vi "Run Program.vi"(0 "Program Path":path=path "%SystemRoot%/System32/calc.exe") -> ()   [LabVIEW 2020]
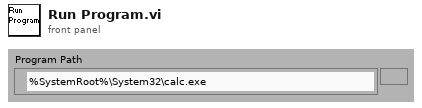
[diagram p1: front panel]
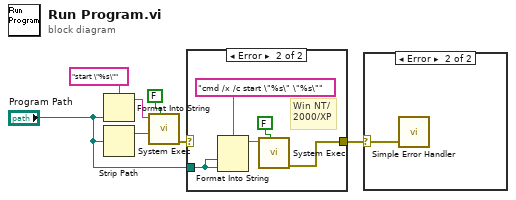
[diagram p0: block diagram]
diagram:
  n1 = Format Into String(format string="start \"%s\"", "Program Path") -> (resulting string=w3:string)  [unwired: 2 in, 1 out]
  n2 = Strip Path(path="Program Path") -> (stripped path=w4:path)  [unwired: 1 out]
  n3 = call <vilib>:"System Exec.vi"("wait until completion? (T)"=FALSE ("Wait until done"), "working directory"=w4, "command line"=w3) -> ("error out"=w5:errorcluster)  [unwired: 5 in, 3 out]
  n4 = case shown="Error" w5 {
    selector: w5 -> [w8 _]
    tunnel: "Program Path" -> [_ w10]
    tunnel: [w8 w9] -> w7
    frame No Error {
    }
    frame Error {
      # "Win NT/\n2000/XP"
      n5 = Format Into String(format string="cmd /x /c start \"%s\" \"%s\"", w10, w10) -> (resulting string=w11:string)  [unwired: 2 in, 1 out]
      n6 = call <vilib>:"System Exec.vi"("wait until completion? (T)"=FALSE ("Wait until done"), "command line"=w11) -> ("error out"=w9:errorcluster)  [unwired: 6 in, 3 out]
    }
  }
  n7 = case shown="Error" w7 {
    selector: w7 -> [_ w14]
    frame No Error {
    }
    frame Error {
      n8 = call <vilib>:"Simple Error Handler.vi"("error in (no error)"=w14) -> ()  [unwired: 4 in, 5 out]
    }
  }
